vi "Interface.vi"(7 "Interface":enum16{"Simulation", "Embedded"}(ring), 8 "Error In":errorcluster) -> (0 "Error Out":errorcluster)   [LabVIEW 2017, in "Controller.lvlib"]
uses:
  Controller.lvlib
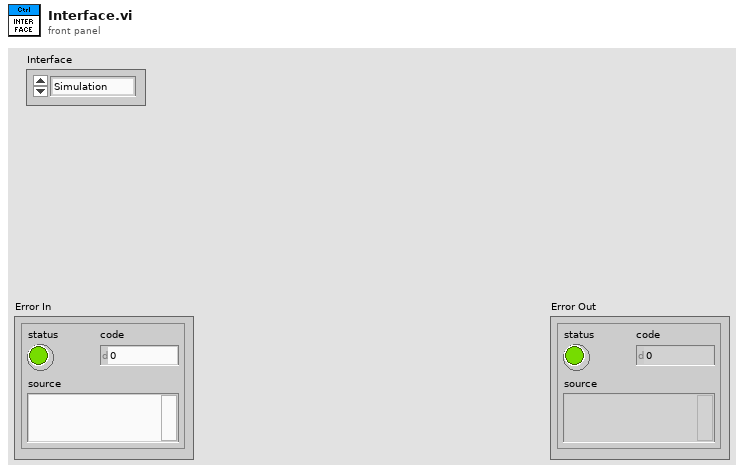
[diagram p1: front panel]
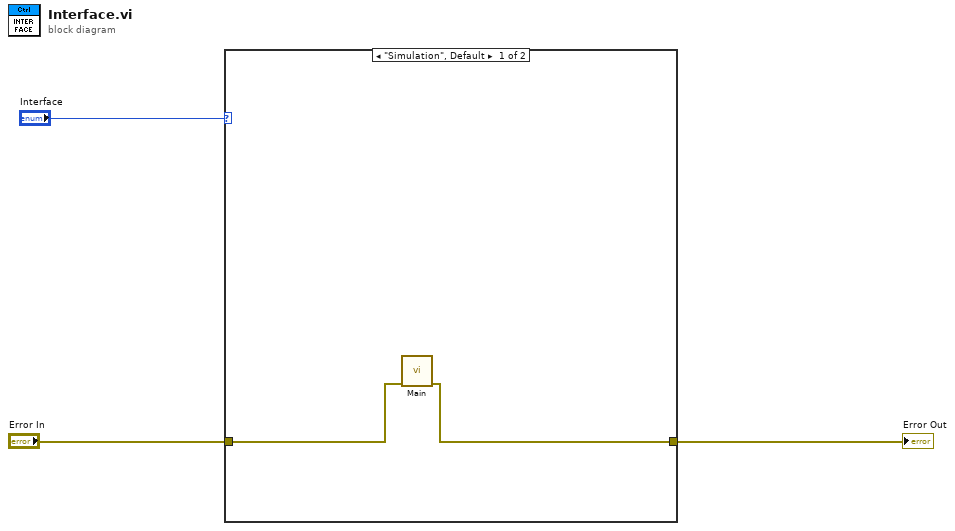
[diagram p0: block diagram]
diagram:
  n1 = case shown="\"Simulation\", Default" "Interface" {
    tunnel: "Error In" -> [w5 w6]
    tunnel: [w4 w6] -> w2
    frame "Simulation", Default {
      n2 = call "Main.vi"("Error In"=w5) -> ("Error Out"=w4:errorcluster)  [unwired: 10 in]
    }
    frame "Embedded" {
    }
  }
  "Error Out" <- w2
